vi "Read Address.lvclass.vi"(8 "error in (no error)":errorcluster, 11 "Speed Mode in":refnum<class "Speed Mode.lvclass">) -> (0 "error out":errorcluster, 2 "Address.lvclass":refnum<class "Address.lvclass">, 3 "Speed Mode out":refnum<class "Speed Mode.lvclass">)   [LabVIEW 2020, in "Speed Mode.lvclass"]
uses:
  Speed Mode.lvclass
  Address/Address.lvclass
  Speed Mode.lvclass/Speed Mode.ctl
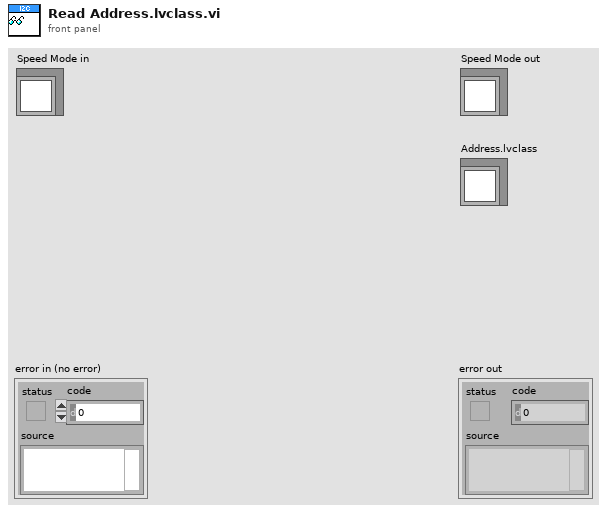
[diagram p1: front panel]
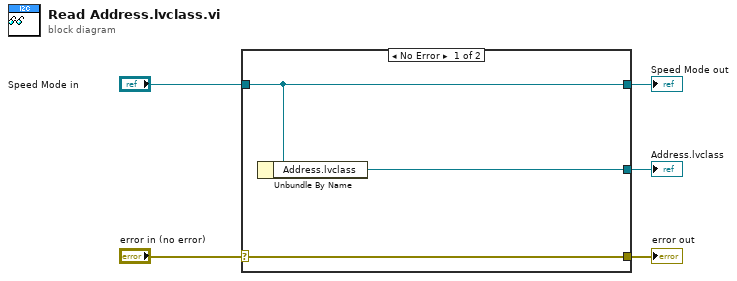
[diagram p0: block diagram]
diagram:
  n1 = case shown="No Error" "error in (no error)" {
    selector: "error in (no error)" -> [w8 w9]
    tunnel: [w8 w9] -> w4
    tunnel: [w7 w10] -> w2
    tunnel: "Speed Mode in" -> [w7 w10]
    tunnel: [w6 _] -> w1
    frame No Error {
      n2 = Unbundle By Name(w7) -> ("Address.lvclass"=w6:refnum<class "Address.lvclass">)
    }
    frame Error {
    }
  }
  "error out" <- w4
  "Speed Mode out" <- w2
  "Address.lvclass" <- w1
